vi "HMF2500 Set Pulse Mode TTL.vi"(8 "error in (no error)":errorcluster, 11 "VISA in":refnum<visa-resource-name>) -> (0 "error out":errorcluster, 3 "VISA out":refnum<visa-resource-name>)   [LabVIEW 2020, in "AWG.lvlib"]
doc: "Set output to pulses with TTL levels and high-Z."
uses:
  AWG.lvlib
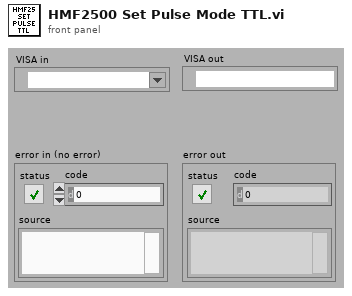
[diagram p1: front panel]
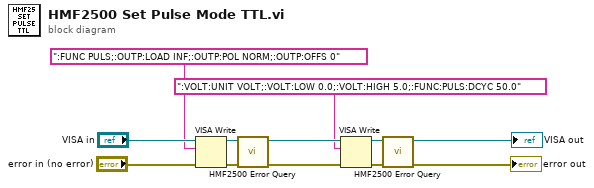
[diagram p0: block diagram]
diagram:
  n1 = VISA Write(VISA resource name="VISA in", write buffer=":FUNC PULS;:OUTP:LOAD INF;:OUTP:POL NORM;:OUTP:OFFS 0", error in (no error)="error in (no error)") -> (VISA resource name out=w8:refnum<visa-resource-name>, error out=w11:errorcluster)  [unwired: 1 out]
  n2 = call "HMF2500 Error Query.vi"("error in (no error)"=w11, "VISA resource name"=w8) -> ("error out"=w5:errorcluster, "VISA resource name out"=w4:refnum<visa-resource-name>)  [unwired: 6 in, 2 out]
  n3 = VISA Write(VISA resource name=w4, write buffer=":VOLT:UNIT VOLT;:VOLT:LOW 0.0;:VOLT:HIGH 5.0;:FUNC:PULS:DCYC 50.0", error in (no error)=w5) -> (VISA resource name out=w7:refnum<visa-resource-name>, error out=w6:errorcluster)  [unwired: 1 out]
  n4 = call "HMF2500 Error Query.vi"("error in (no error)"=w6, "VISA resource name"=w7) -> ("error out"=→"error out":errorcluster, "VISA resource name out"=→"VISA out":refnum<visa-resource-name>)  [unwired: 6 in, 2 out]
